vi "Flight Gear Interface Initialization VI.vi"(8 "error in (no error)":errorcluster, 10 "Custom XML":string, 11 "Device Item Ref in":T3 format="%.0x") -> (0 "error out":errorcluster, 3 "Device Item Ref out":T3 format="%.0x")   [LabVIEW 2010, in "Flight Gear Interface Custom Device.lvlib"]
uses:
  Flight Gear Interface Custom Device.lvlib
  <vilib>/NI VeriStand/Custom Device API/Custom Device Item Ref.ctl
  <vilib>/NI VeriStand/Custom Device API/Custom Device Channel.ctl
  <vilib>/NI VeriStand/Custom Device API/Custom Device Channel Type.ctl
  <vilib>/NI VeriStand/Custom Device API/Custom Device Timed Loop Priority.ctl
  <vilib>/NI VeriStand/Custom Device API/Custom Device Loop Type.ctl
  <vilib>/NI VeriStand/Custom Device API/Set Item Property (String).vi
  <vilib>/NI Veristand/Custom Device API/Custom Device API.lvlib
panel:
  in  "Channel":T1={"Type"=enum."Input", "Units"="", "Default Value"=0.0, "Faultable"=TRUE, "Scalable"=TRUE}
  in  "Channels":string[](array[string])=["Airspeed", "Phi", "Theta", "Psi", "Longitude", "Latitude", "Altitude"]
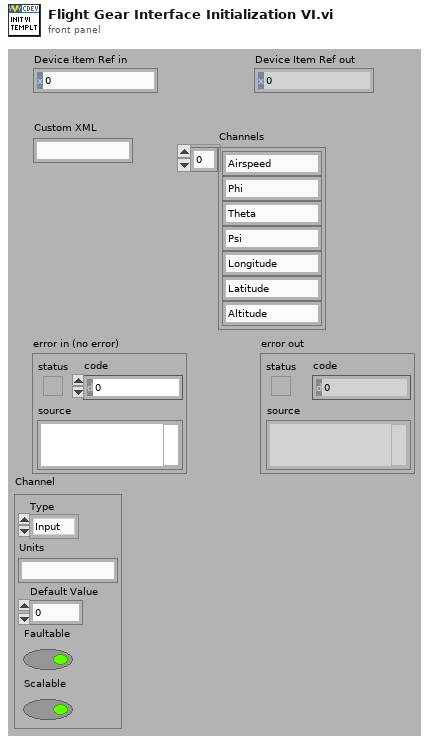
[diagram p1: front panel]
types:
  T1 = typedef "Custom Device API.lvlib/Custom Device Channel.ctl" = cluster{"Type":T2, "Units":string, "Default Value":dbl, "Faultable":bool, "Scalable":bool}
  T2 = typedef "Custom Device API.lvlib/Custom Device Channel Type.ctl" = enum16{"Input", "Output"}
  T3 = typedef "Custom Device API.lvlib/Custom Device Item Ref.ctl" = u64
  T4 = typedef "Custom Device API.lvlib/Custom Device Timed Loop Priority.ctl" = enum32{"Low", "Medium", "High"}
  T5 = typedef "Custom Device API.lvlib/Custom Device Loop Type.ctl" = enum32{"While Loop", "Timed Loop"}
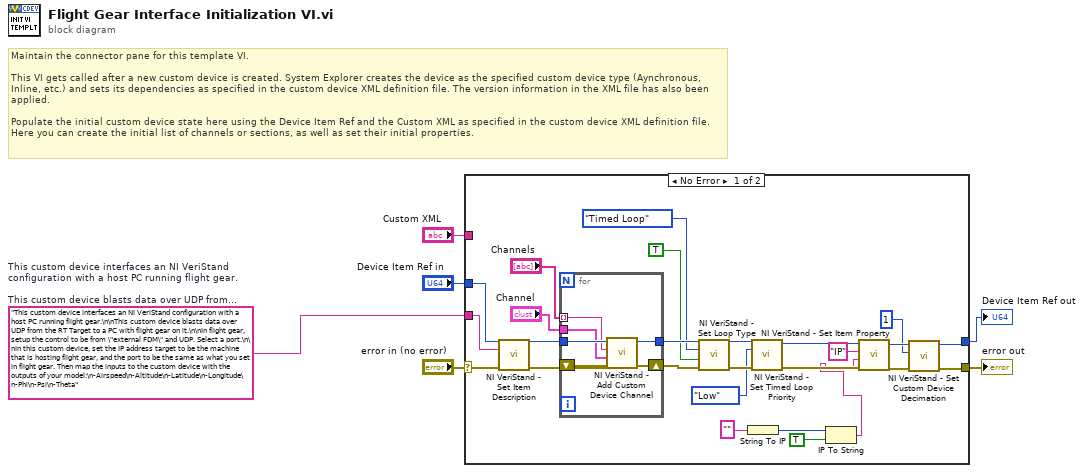
[diagram p0: block diagram]
diagram:
  w1 = "This custom device interfaces an NI VeriStand configuration with a host PC running flight gear.\n\nThis custom device blasts data over UDP from the RT Target to a PC with flight gear on it.\n\nIn flight gear, setup the control to be from \"external FDM\" and UDP. Select a port.\n\nIn this custom device, set the IP address target to be the machine that is hosting flight gear, and the port to be the same as what you set in flight gear. Then map the inputs to the custom device with the outputs of your model:\n-Airspeed\n-Altitude\n-Latitude\n-Longitude\n-Phi\n-Psi\n-Theta"  # This custom device interfaces an NI VeriStand configuration with a host PC running flight gear.  This custom device blasts data over UDP from the RT Target to a PC with flight gear on it.  In flight gear, setup the control to be from "external FDM" and UDP. Select a port.  In this custom device, set the IP address target to be the machine that is hosting flight gear, and the port to be the same as what you set in flight gear. Then map the inputs to the custom device with the outputs of your model: -Airspeed -Altitude -Latitude -Longitude -Phi -Psi -Theta
  # "Maintain the connector pane for this template VI.\n\nThis VI gets called after a new custom device is created. System Explorer creates the device as the specified custom device type (Aynchronous, Inline, etc.) and sets its dependencies as specified in the custom device XML definition file. The version information in the XML file has also been applied.\n\nPopulate the initial custom device state here using the Device Item Ref and the Custom XML as specified in the custom device XML definition file. Here you can create the initial list of channels or sections, as well as set their initial properties."
  n1 = case shown="No Error" "error in (no error)" {
    selector: "error in (no error)" -> [w31 w40]
    tunnel: [w11 w40] -> w6
    tunnel: [w10 w39] -> w4
    tunnel: "Device Item Ref in" -> [w32 w39]
    tunnel: "Custom XML" -> [_ _]
    tunnel: w1 -> [w30 _]
    frame No Error {
      n2 = call <vilib>:"NI VeriStand - Set Item Description.vi"("error in (no error)"=w31, "Description"=w30, "Item Ref in"=w32) -> ("error out"=w29:errorcluster, "Item Ref out"=w28:T3)  [unwired: 6 in, 1 out]
      n3 = for {
        tunnel: w28 -> [w37]
        tunnel: "Channels" -> [w36] mode=indexing
        tunnel: "Channel" -> [w35]
        shift-right: [w34] -> w25
        shift-left: w29 -> [w38]
        tunnel: [w33] -> w24
        n4 = call <vilib>:"NI VeriStand - Add Custom Device Channel.vi"("error in (no error)"=w38, "Channel"=w35, "Channel Name"=w36, "Parent Ref in"=w37) -> ("error out"=w34:errorcluster, "Parent Ref out"=w33:T3)  [unwired: 4 in, 2 out]
      }
      n5 = call <vilib>:"NI VeriStand - Set Loop Type.vi"("error in (no error)"=w25, "Use Device Clock (Timed Loops only)"=TRUE, "Loop type"=Custom_Device_Loop_Type."Timed Loop", "Device Ref in"=w24) -> ("error out"=w21:errorcluster, "Device Ref out"=w20:T3)  [unwired: 6 in]
      n6 = String To IP(1:"" ("name")) -> (0:w14:u32)
      n7 = call <vilib>:"NI VeriStand - Set Timed Loop Priority.vi"("error in (no error)"=w21, "Priority"=Custom_Device_Timed_Loop_Priority."Low", "Device Ref in"=w20) -> ("error out"=w18:errorcluster, "Device Ref out"=w17:T3)  [unwired: 7 in]
      n8 = IP To String(1:TRUE ("dot notation? (F)"), 2:w14) -> (0:w12:string)
      n9 = call-poly <vilib>:"NI VeriStand - Set Item Property.vi"("error in (no error)"=w18, "Value"=w12, "Property Name"="IP", "Item Ref in"=w17) -> ("error out"=w8:errorcluster, "Item Ref out"=w9:T3)  [unwired: 5 in, 1 out]
      n10 = call <vilib>:"NI VeriStand - Set Custom Device Decimation.vi"("error in (no error)"=w8, "Decimation"=1, "Device Ref in"=w9) -> ("error out"=w11:errorcluster, "Device Ref out"=w10:T3)  [unwired: 7 in]
    }
    frame Error {
    }
  }
  "error out" <- w6
  "Device Item Ref out" <- w4
